vi "Temperature Monitor.vi"() -> ()   [LabVIEW 2015]
doc: "This VI is the solution to an exercise in the LabVIEW Core 1 course.\n\nIt uses a While Loop and shift registers to average data. No hardware is necessary."
panel:
  in  "Num Elements\nto Average":i32=10
  in  "Delay in ms":u32=10
  in  "Stop Button":bool
  out "Temperature History":dbl(graph)=30.425781249999993
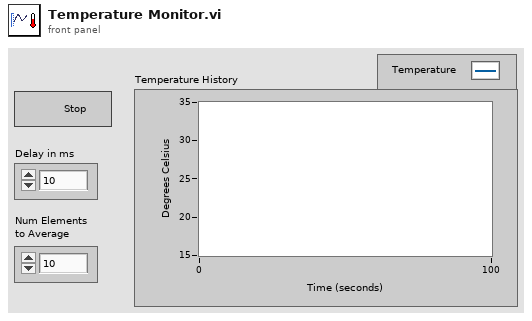
[diagram p1: front panel]
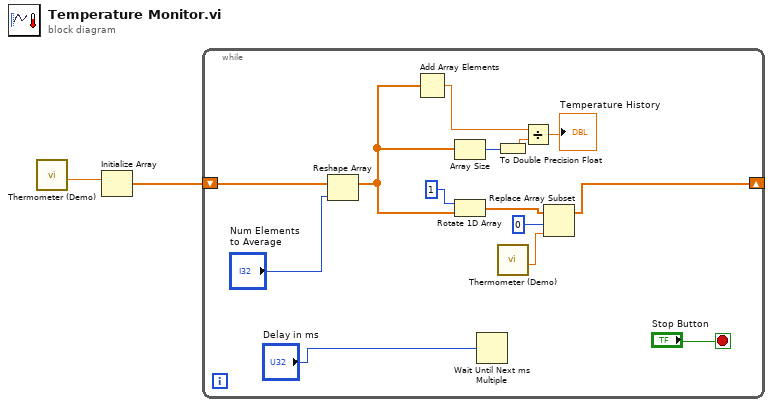
[diagram p0: block diagram]
diagram:
  n1 = call "Thermometer (Demo).vi"() -> ("Temperature Value"=w2:dbl)  [unwired: 11 in]
  n2 = Initialize Array(w2) -> (w1:dbl[])  [unwired: 1 in]
  n3 = while {
    shift-right: [w4] -> _
    shift-left: w1 -> [w10]
    stop <- "Stop Button" stop-if-true
    n4 = Reshape Array(w10, "Num Elements\nto Average") -> (w8:dbl[])
    n5 = Add Array Elements(numeric array=w8) -> (sum=w11:dbl)
    n6 = Array Size(array=w8) -> (size(s)=w12:i32)
    n7 = Rotate 1D Array(1:w8, 2:1) -> (0:w6:dbl[])
    n8 = Wait Until Next ms Multiple(millisecond multiple="Delay in ms") -> ()  [unwired: 1 out]
    n9 = To Double Precision Float(number=w12) -> (double precision float=w15:dbl)
    n10 = call "Thermometer (Demo).vi"() -> ("Temperature Value"=w5:dbl)  [unwired: 11 in]
    n11 = Divide(x=w11, y=w15) -> (x/y=→"Temperature History":dbl)
    n12 = Replace Array Subset(array=w6, new element=w5, index=0) -> (w4:dbl[])
  }
